vi "LVITX Format string 1D.vi"(1 "X 1D Array":string[](array[string]), 2 "X  Array name":string) -> (0 "String":string)   [LabVIEW 2016, in "LVtoITX.lvclass"]
uses:
  LVtoITX.lvclass
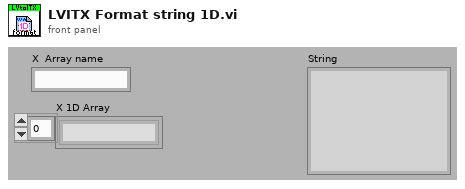
[diagram p1: front panel]
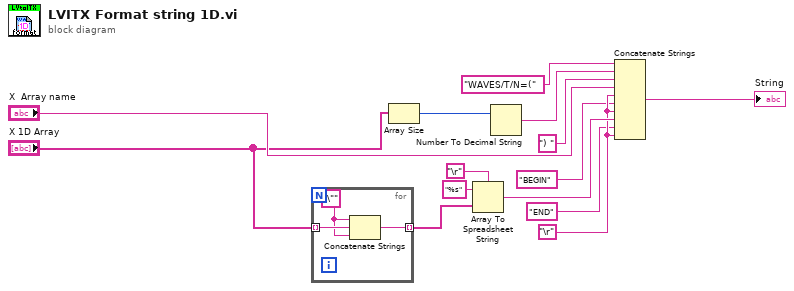
[diagram p0: block diagram]
diagram:
  w8 = "\r"
  n1 = for {
    tunnel: "X 1D Array" -> [w17] mode=indexing
    tunnel: [w16] -> w1 mode=indexing
    w15 = "\"" ("string")
    n2 = Concatenate Strings(w15, w17, w15) -> (w16:string)
  }
  n3 = Array Size(array="X 1D Array") -> (size(s)=w3:i32)
  n4 = Array To Spreadsheet String(delimiter (Tab)="\r", array=w1, 3:"%s" ("format string")) -> (spreadsheet string=w9:string)
  n5 = Number To Decimal String(number=w3) -> (decimal integer string=w11:string)  [unwired: 1 out]
  n6 = Concatenate Strings("WAVES/T/N=(", w11, ") ", "X  Array name", w8, "BEGIN", w8, w9, "END", w8) -> (→"String":string)
